vi "SPIFreSet.vi"(8 "error in (no error)":errorcluster caption="错误输入（无错误）", 10 "Frequency(Hz)":i32(ring)=400 items=["1"=1, "10"=10, "40"=40, "100"=100, "400"=400, "1000"=1000, "4000"=4000, "10000"=10000, "40000"=40000, "100000"=100000, "400000"=400000, "1000000"=1000000, "4000000"=4000000, "10000000"=10000000], 11 "handle":u64) -> (0 "error out":errorcluster caption="错误输出", 2 "function return":i32, 3 "handle out":u64)   [LabVIEW 2018]
doc: "s"
uses:
  InstrumentsPlayground.lvlib
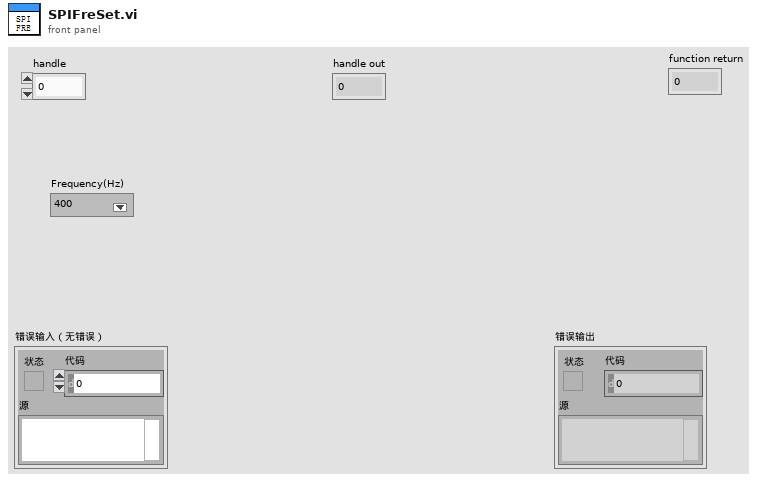
[diagram p1: front panel]
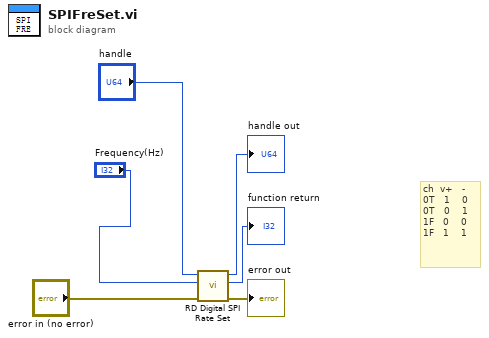
[diagram p0: block diagram]
diagram:
  # "ch  v+   -\n0T   1    0\n0T   0    1\n1F   0    0\n1F   1    1"
  n1 = call "RD Digital SPI Rate Set.vi"("error in (no error)"="error in (no error)", "rate"="Frequency(Hz)", "handle"="handle") -> ("error out"=→"error out":errorcluster, "function return"=→"function return":i32, "handle out"=→"handle out":u64)  [unwired: 6 in]
